vi "VI Pop Up Backup.vi"(7 "Aufrufer gesperrt?":bool, 8 "Fehler (Eingang, kein Fehler)":errorcluster, 11 "VI Referenz":refnum<vi>) -> (0 "Fehler (Ausgang)":errorcluster, 3 "Referenz (Ausgang)":refnum<vi>)   [LabVIEW 2015, in "Backup.lvlib"]
uses:
  Backup.lvlib
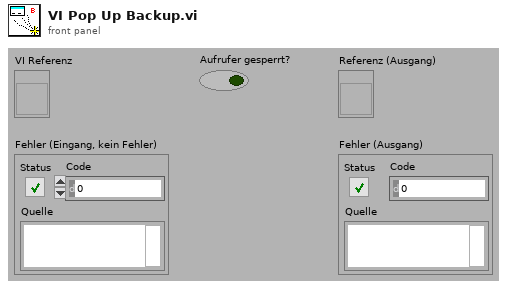
[diagram p1: front panel]
types:
  T1 = enum32{"Bad", "Idle", "Run top level", "Running"}
  T2 = enum32{"Invalid", "Default", "Floating", "Floating/Auto-Hide", "Modal"}
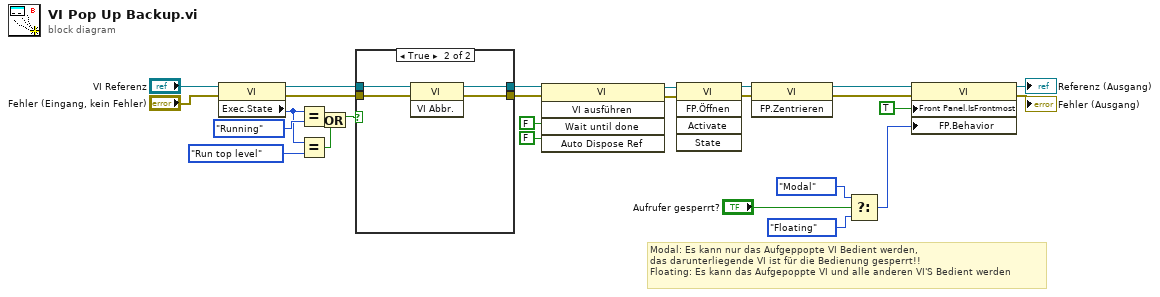
[diagram p0: block diagram]
diagram:
  # "Modal: Es kann nur das Aufgeppopte VI Bedient werden, \ndas darunterliegende VI ist für die Bedienung gesperrt!!\nFloating: Es kann das Aufgepoppte VI und alle anderen VI'S Bedient werden"
  n1 = property class="VI"(reference="VI Referenz", error in="Fehler (Eingang, kein Fehler)") -> (reference out=w11:refnum<vi>, error out=w9:errorcluster, "Exec.State"=w7:T1)
  n2 = Equal?(x=w7, y=T1."Running" ("Ausführung:Status")) -> (x = y?=w10:bool)
  n3 = Equal?(x=w7, y=T1."Run top level" ("Ausführung:Status")) -> (x = y?=w5:bool)
  n4 = Or(x=w10, y=w5) -> (x .or. y?=w6:bool)
  n5 = case shown="True" w6 {
    tunnel: w11 -> [w29 w33]
    tunnel: [w29 w32] -> w2
    tunnel: w9 -> [w28 w31]
    tunnel: [w28 w30] -> w1
    frame False {
    }
    frame True {
      n6 = invoke class="VI" method="VI Abbr."(reference=w33, error in=w31) -> (reference out=w32:refnum<vi>, error out=w30:errorcluster)  [unwired: 1 in, 1 out]
    }
  }
  n7 = invoke class="VI" method="VI ausführen"(reference=w2, error in=w1, "Wait until done"=FALSE ("Warten bis beendet"), "Auto Dispose Ref"=FALSE ("Referenz automatisch schließen")) -> (reference out=w25:refnum<vi>, error out=w24:errorcluster)  [unwired: 1 in, 3 out]
  n8 = invoke class="VI" method="FP.Öffnen"(reference=w25, error in=w24) -> (reference out=w23:refnum<vi>, error out=w22:errorcluster)  [unwired: 3 in, 3 out]
  n9 = invoke class="VI" method="FP.Zentrieren"(reference=w23, error in=w22) -> (reference out=w15:refnum<vi>, error out=w21:errorcluster)  [unwired: 1 in, 1 out]
  n10 = Select(t=T2."Modal" ("Frontpanel-Fenster:Verhaltensweise"), s="Aufrufer gesperrt?", f=T2."Floating" ("Frontpanel-Fenster:Verhaltensweise")) -> (s? t:f=w16:T2)
  n11 = property class="VI"(reference=w15, error in=w21, "Front Panel.IsFrontmost"=TRUE ("Frontpanel-Fenster:Ist im Vordergrund"), "FP.Behavior"=w16) -> (reference out=→"Referenz (Ausgang)":refnum<vi>, error out=→"Fehler (Ausgang)":errorcluster)
